vi "SMO.jsonRPC.SendSynchronousCommand.vi"(7 "Notification":bool, 8 "error in (no error)":errorcluster, 9 "Parameters":variant, 10 "Method":string, 11 "SMO.jsonRPC in":refnum<class "SMO.jsonRPC.lvclass">) -> (0 "error out":errorcluster, 2 "id":i32, 3 "SMO.jsonRPC out":refnum<class "SMO.jsonRPC.lvclass">)   [LabVIEW 2013, in "SMO.jsonRPC.lvclass"]
uses:
  SMO.jsonRPC.lvclass
  Typedefs/Request--Cluster.ctl
  <vilib>/JKI/JKI JSON RPC Specification/Request/Request.lvclass
  <vilib>/JKI/JKI JSON RPC Specification/Response/Response.lvclass
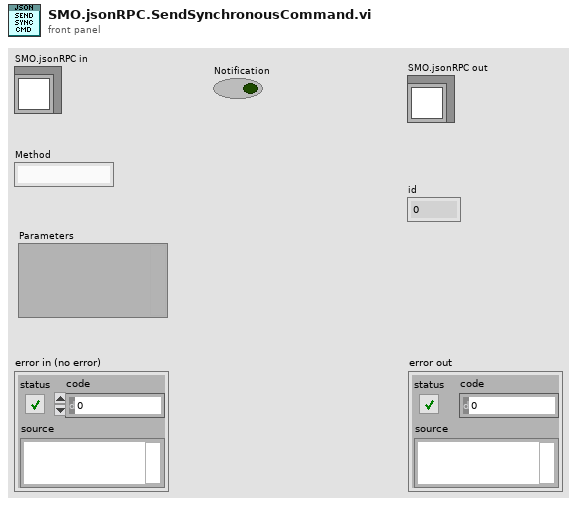
[diagram p1: front panel]
types:
  T1 = typedef "SMO.jsonRPC.lvclass/Request--Cluster.ctl" = cluster{"Request":refnum<class "Request.lvclass">, "reply queue":refnum<queue>, "Async?":bool}
  T2 = typedef "SMO.jsonRPC.lvclass/PrivateEvents--Cluster.ctl" = cluster{"Incoming Request":refnum<user-event>}
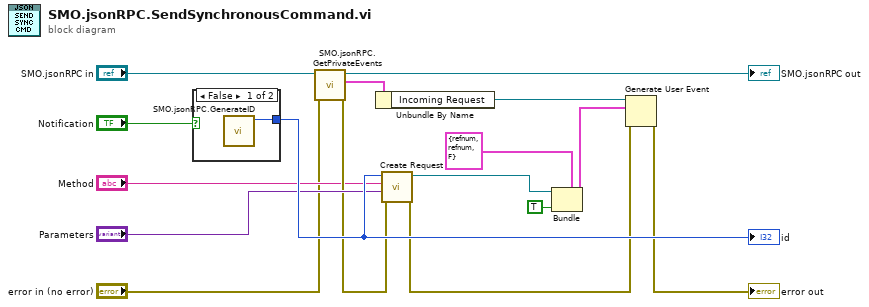
[diagram p0: block diagram]
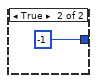
[diagram p2: hidden frame]
diagram:
  n1 = case shown="False" "Notification" {
    tunnel: [w17 -1 ("id")] -> w15
    frame False {
      n2 = call "SMO.jsonRPC.GenerateID.vi"() -> ("id"=w17:i32)  [unwired: 11 in]
    }
    frame True {
    }
  }
  "id" <- w15
  n3 = call "SMO.jsonRPC.GetPrivateEvents.vi"("error in (no error)"="error in (no error)", "SMO.jsonRPC"="SMO.jsonRPC in") -> ("error out"=w12:errorcluster, "Private Events"=w5:T2, "SMO.jsonRPC out"=→"SMO.jsonRPC out":refnum<class "SMO.jsonRPC.lvclass">)  [unwired: 7 in]
  n4 = Unbundle By Name(w5) -> ("Incoming Request"=w4:refnum<user-event>)
  n5 = call <vilib>:"Create Request.vi"("error in (no error)"=w12, "Parameters"="Parameters", "Method"="Method", "id (-1: notification)"=w15) -> ("error out"=w13:errorcluster, "Request"=w10:refnum<class "Request.lvclass">)  [unwired: 5 in, 1 out]
  n6 = Bundle(cluster=T1 {"Request"=refnum, "reply queue"=refnum, "Async?"=FALSE} ("event data"), "Request"=w10, "Async?"=TRUE) -> (w7:T1)  [unwired: 1 in]
  n7 = Generate User Event(user event=w4, event data cluster=w7, error in=w13) -> (error out=→"error out":errorcluster)  [unwired: 1 in, 1 out]
